vi "Exp PDF.vi"(9 "b":dbl=1.0, 10 "a":dbl, 11 "x":dbl=1.0) -> (0 "error":i32, 3 "pdf(x)":dbl=0.36787944117144233)   [LabVIEW 2014, in "NI_Gmath.lvlib"]
doc: "Computes the continuous probability density function (PDF) of various distributions. You must manually select the polymorphic instance to use."
uses:
  NI_Gmath.lvlib
  st_error_code.ctl
panel:
  # "Exp PDF"
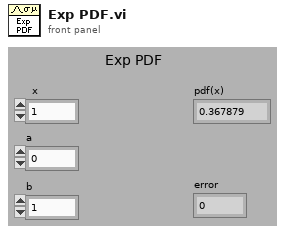
[diagram p1: front panel]
types:
  T1 = typedef "NI_Gmath.lvlib/st_error_code.ctl" = i32
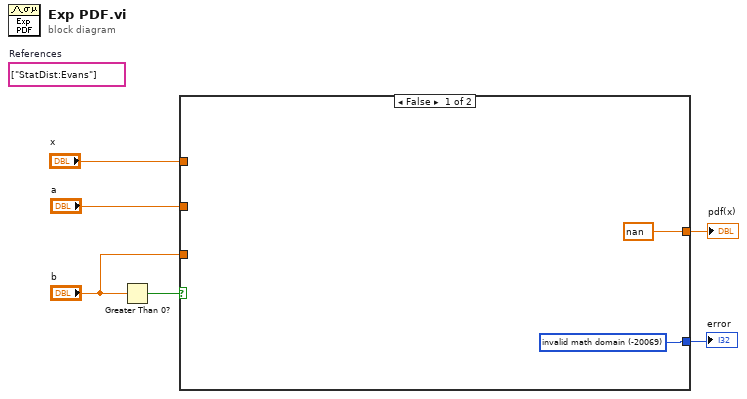
[diagram p0: block diagram]
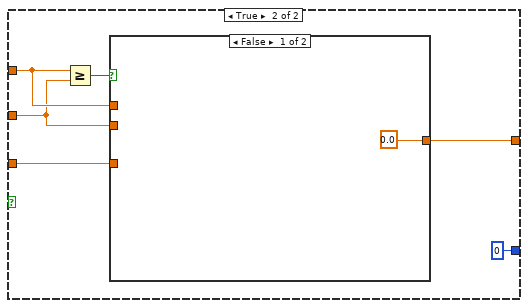
[diagram p2: hidden frame]
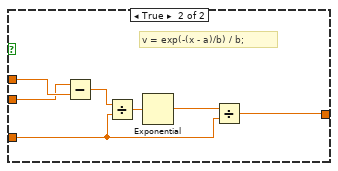
[diagram p3: hidden frame]
diagram:
  (unwired) string[] ["StatDist:Evans"]  # References
  n1 = Greater Than 0?(x="b") -> (x > 0?=w2:bool)
  n2 = case shown="False" w2 {
    tunnel: "b" -> [_ w12]
    tunnel: [w7 0 ("invalid math domain")] -> w6
    tunnel: [nan w13] -> w5
    tunnel: "x" -> [_ w10]
    tunnel: "a" -> [_ w9]
    frame False {
      w7 = T1 -20069 items=["invalid math domain"=-20069, "Fourier interpolation size m >= n"=-20070, "empty array"=-20003] ("stat interp error code")
    }
    frame True {
      n3 = Greater Or Equal?(x=w10, y=w9) -> (x >= y?=w11:bool)
      n4 = case shown="False" w11 {
        tunnel: [0.0 w16] -> w13
        tunnel: w10 -> [_ w22]
        tunnel: w9 -> [_ w21]
        tunnel: w12 -> [_ w18]
        frame False {
        }
        frame True {
          # "v = exp(-(x - a)/b) / b;"
          n5 = Subtract(x=w21, y=w22) -> (x-y=w20:dbl)
          n6 = Divide(x=w20, y=w18) -> (x/y=w19:dbl)
          n7 = Exponential(1:w19) -> (0:w17:dbl)
          n8 = Divide(x=w17, y=w18) -> (x/y=w16:dbl)
        }
      }
    }
  }
  "pdf(x)" <- w5
  "error" <- w6
